vi "Finger_Calibration.vi"(7 "Calibrate?":bool, 8 "Hand Position":cluster{"X":dbl, "Y":dbl, "Z":dbl}, 9 "Finger Positions":T1(array[cluster]), 10 "Max distance in":dbl[](array[numeric]), 11 "Not Tracked?":bool) -> (3 "Max distance out":dbl[](array[numeric]))   [LabVIEW 2015]
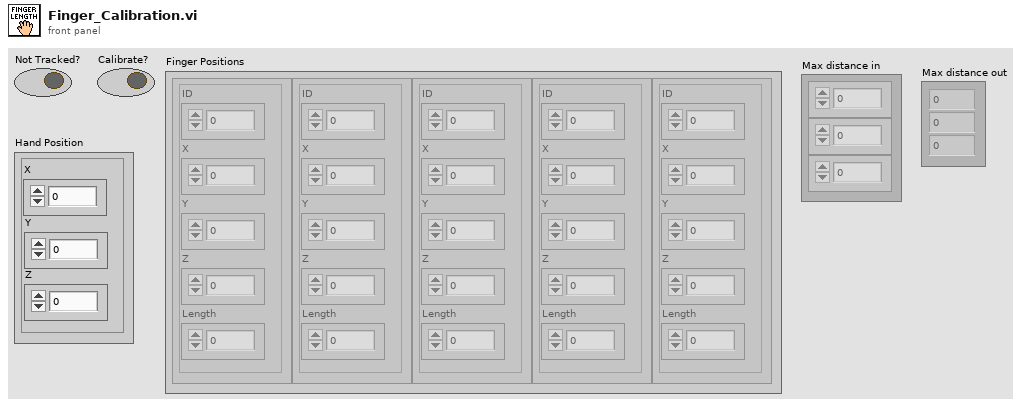
[diagram p1: front panel]
types:
  T1 = cluster{"ID":dbl, "X":dbl, "Y":dbl, "Z":dbl, "Length":dbl}[]
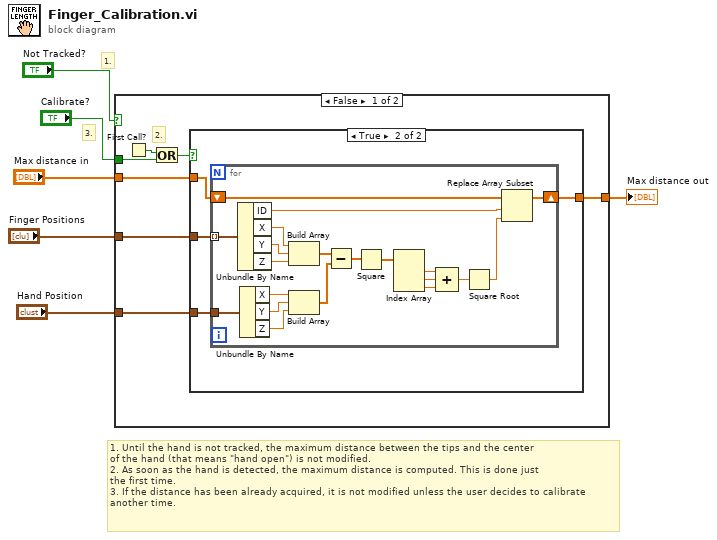
[diagram p0: block diagram]
diagram:
  # "3."
  # "1."
  # "1. Until the hand is not tracked, the maximum distance between the tips and the center \nof the hand (that means \"hand open\") is not modified.\n2. As soon as the hand is detected, the maximum distance is computed. This is done just \nthe first time.\n3. If the distance has been already acquired, it is not modified unless the user decides to calibrate\nanother time."
  n1 = case shown="False" "Not Tracked?" {
    tunnel: "Finger Positions" -> [w13 _]
    tunnel: "Hand Position" -> [w12 _]
    tunnel: [w11 w39] -> w6
    tunnel: "Max distance in" -> [w10 w39]
    tunnel: "Calibrate?" -> [w7 _]
    frame False {
      # "2."
      n2 = First Call?() -> (First Call?: T/F=w9:bool)
      n3 = Or(x=w9, y=w7) -> (x .or. y?=w8:bool)
      n4 = case shown="True" w8 {
        tunnel: w13 -> [_ w18]
        tunnel: w12 -> [_ w17]
        tunnel: [w14 w15] -> w11
        tunnel: w10 -> [w14 w16]
        frame False {
        }
        frame True {
          n5 = for {
            tunnel: w18 -> [w36] mode=indexing
            tunnel: w17 -> [w35]
            shift-right: [w19] -> w15
            shift-left: w16 -> [w20]
            n6 = Unbundle By Name(w36) -> ("ID"=w21:dbl, "X"=w34:dbl, "Y"=w33:dbl, "Z"=w32:dbl)
            n7 = Unbundle By Name(w35) -> ("X"=w31:dbl, "Y"=w30:dbl, "Z"=w29:dbl)
            n8 = Build Array(w34, w33, w32) -> (w28:dbl[])
            n9 = Build Array(w31, w30, w29) -> (w27:dbl[])
            n10 = Subtract(x=w28, y=w27) -> (x-y=w38:dbl[])
            n11 = Square(x=w38) -> (x^2=w26:dbl[])
            n12 = Index Array(array=w26) -> (element #1=w25:dbl, element #2=w24:dbl, element #3=w23:dbl)  [unwired: 3 in]
            n13 = Compound Arithmetic op=ADD(w25, w24, w23) -> (w37:dbl)
            n14 = Square Root(x=w37) -> (sqrt(x)=w22:dbl)
            n15 = Replace Array Subset(array=w20, new element=w22, index=w21) -> (w19:dbl[])
          }
        }
      }
    }
    frame True {
    }
  }
  "Max distance out" <- w6
